vi "runningaverage.vi"(9 "Iteration":i32, 10 "New value":dbl, 11 "Average in":dbl) -> (3 "Average out":dbl)   [LabVIEW 2010]
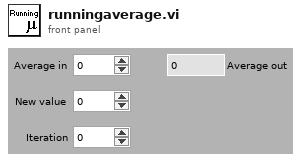
[diagram p1: front panel]
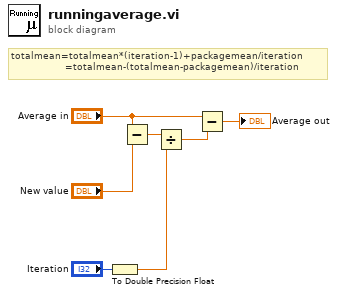
[diagram p0: block diagram]
diagram:
  # "totalmean=totalmean*(iteration-1)+packagemean/iteration\n                  =totalmean-(totalmean-packagemean)/iteration"
  n1 = To Double Precision Float(number="Iteration") -> (double precision float=w4:dbl)
  n2 = Subtract(x="Average in", y="New value") -> (x-y=w6:dbl)
  n3 = Divide(x=w6, y=w4) -> (x/y=w2:dbl)
  n4 = Subtract(x="Average in", y=w2) -> (x-y=→"Average out":dbl)
